vi "VSI Slave Write Bytes.vi"(7 "WriteBytesNum":i32, 9 "pWriteData":u8[](array[numeric])=array[10240 elements], 10 "DevIndex":i32, 11 "DevType":i32) -> (3 "function return":i32)   [LabVIEW 2010, in "ControlSPI.lvlib"]
doc: "int WINAPI VSI_SlaveWriteBytes(int DevType,int DevIndex,unsigned char *pWriteData,int WriteBytesNum);"
uses:
  ControlSPI.lvlib
  ControlSPI/Ginkgo_Driver.dll
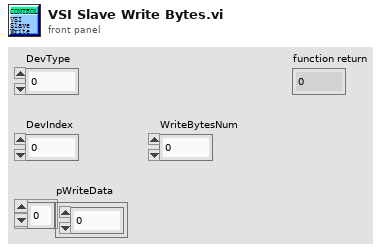
[diagram p1: front panel]
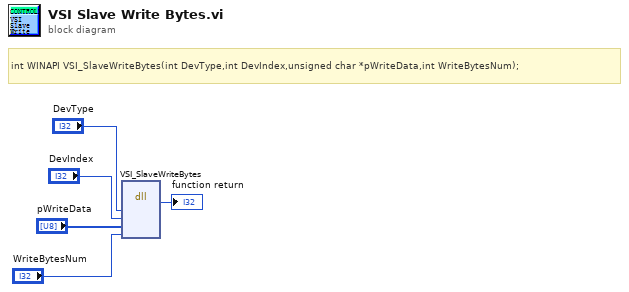
[diagram p0: block diagram]
diagram:
  # "int WINAPI VSI_SlaveWriteBytes(int DevType,int DevIndex,unsigned char *pWriteData,int WriteBytesNum);"
  n1 = dll-call lib="E:/Project/vt_ginkgo/truck/Ginkgo Driver/vs2010/Ginkgo_USB-I2C&SPI&CAN_API_v2.0.3.3/lib/labview_32bit/ControlSPI/Ginkgo_Driver.*" fn="VSI_SlaveWriteBytes"("DevType"="DevType", "DevIndex"="DevIndex", "pWriteData"="pWriteData", "WriteBytesNum"="WriteBytesNum") -> (→"function return":i32)  [unwired: 7 in, 2 out]
